vi "Close.vi"(8 "error in (no error)":errorcluster, 11 "VISA resource name":refnum<visa-resource-name>) -> (0 "error out":errorcluster)   [LabVIEW 2019, in "KH7008.lvlib"]
uses:
  KH7008.lvlib
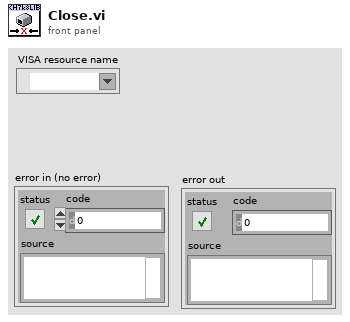
[diagram p1: front panel]
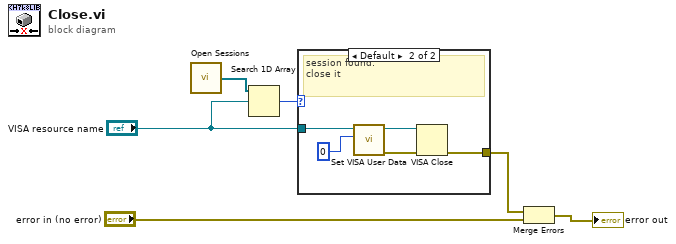
[diagram p0: block diagram]
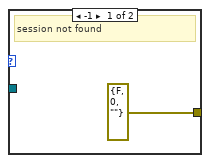
[diagram p2: hidden frame]
diagram:
  n1 = call <vilib>:"Open Sessions.vi"() -> ("Array of Refnums"=w4:refnum<visa-resource-name>[])  [unwired: 2 in]
  n2 = Search 1D Array(1D array=w4, element="VISA resource name") -> (index of element=w2:i32)  [unwired: 1 in]
  n3 = case shown="Default" w2 {
    tunnel: "VISA resource name" -> [_ w11]
    tunnel: [errorcluster {"status"=FALSE, "code"=0, "source"=""} ("error out") w12] -> w3
    frame -1 {
      # "session not found"
    }
    frame Default {
      # "session found:\nclose it"
      n4 = call "Set VISA User Data.vi"("User Data"=0, "VISA Refnum in"=w11) -> ("error out"=w8:errorcluster, "VISA Refnum out"=w10:refnum<visa-resource-name>)  [unwired: 8 in]
      n5 = VISA Close(VISA resource name=w10, error in (no error)=w8) -> (error out=w12:errorcluster)
    }
  }
  n6 = Merge Errors(w3, "error in (no error)") -> (→"error out":errorcluster)
